vi "Prepare Acquired Waveforms for Parsing.vi"(4 "append virtual reference":bool, 6 "propagation delay":T1, 7 "restart (F)":bool, 8 "error in":errorcluster, 9 "SV Signal":refnum<class "SV Signal.lvclass">, 10 "tolerance":dbl=0.1 format="%#_13g", 11 "acquired channel waveforms":waveform(dbl)[](array[waveform])) -> (0 "error out":errorcluster, 3 "aligned channel waveforms":waveform(dbl)[](array[waveform]), 5 "alignment reference detected":bool)   [LabVIEW 2022 SP3]
doc: "Align signals and optionally append virtual reference prior to writing data to SV Buffer and parsing for measurement samples."
uses:
  <vilib>/addons/_NISVFA/_Generation/Signal Generation/SV Signal/SV Signal.lvclass
  <vilib>/addons/_NISVFA/_Generation/Signal Generation/SV Signal/SV Signal.lvclass/SV Signal.ctl
  <vilib>/addons/_NISVFA/_Generation/Signal Generation/SV Signal/Read Synchronization Pulse Waveform.vi
  Program Files/NI/LVAddons/nisvt/1/examples/Sound and Vibration/Audio Measurements/subVIs/sv_Measure Delay for Active and Idle Channels.vi
  <vilib>/addons/_NISVFA/_Generation/Signal Generation/SV Signal/Read Leading Synchronization Pulse Enable.vi
  <vilib>/addons/_NISVFA/_Generation/Signal Generation/SV Signal/Read Trailing Synchronization Pulse Enable.vi
  <vilib>/addons/_NISVFA/_Generation/Signal Generation/SV Signal/Write Leading Synchronization Pulse Enable.vi
  <vilib>/addons/_NISVFA/_Shared subVIs/Common/svc_Check for Waveform Parameter Continuity (no state).vi
  <vilib>/addons/_NISVFA/_Shared subVIs/Common/sv_Get NI Property Name String.vi
  <vilib>/addons/Sound and Vibration/svt_Calibration/SV Measure Delay and Polarity and Coherence (Nx1).vi
  Program Files/NI/LVAddons/nisvt/1/examples/Sound and Vibration/Audio Measurements/subVIs/sv_Assign Delay to Idle Channels.vi
  <vilib>/addons/_NISVFA/_Shared subVIs/Common/svc_Get SV Channel Info.vi
  <vilib>/addons/Sound and Vibration/svt_Calibration/SV Measure Delay and Polarity and Coherence.vi
  <vilib>/addons/_NISVFA/_Shared subVIs/Common/svc_Unit Label to Engineering Units.vi
  <vilib>/addons/_NISVFA/_Shared subVIs/Common/svc_Engineering Units to Unit Label.vi
  <vilib>/Analysis/_algsub.llb/Vector Norm.vi
  <vilib>/Analysis/_algsub.llb/Real Vector Norm.vi
  <vilib>/addons/_NISVFA/_Shared subVIs/Common/SV Get Data Subset.vi
  <vilib>/addons/_NISVFA/_Shared subVIs/Common/svc_Get Array Subset (Index).vi
  <vilib>/addons/_NISVFA/_Shared subVIs/Common/svc_Coerce Index and Length.vi
  <vilib>/addons/_NISVFA/_Shared subVIs/Common/svc_Conditional Merge Error.vi
  <vilib>/addons/_NISVFA/_Generation/Signal Generation/SV Signal/Read System Timing Model.vi
  <vilib>/addons/_NISVFA/_Generation/Signal Generation/SV Signal/Write System Timing Model.vi
  <vilib>/addons/_NISVFA/_Shared subVIs/Data Objects/Waveforms (DBL)/Write to Buffer.vi
  <vilib>/addons/_NISVFA/_Shared subVIs/Data Objects/Waveforms (DBL)/Read from Buffer.vi
  <vilib>/addons/_NISVFA/_Shared subVIs/Data Objects/Waveforms (DBL)/SV Read Newest Data.vi
  <vilib>/measure/maresamp.llb/Resample Waveforms (single shot).vi
  <vilib>/measure/maresamp.llb/Resample Waveform (single shot).vi
  <vilib>/addons/_NISVFA/_Shared subVIs/Common/svc_Check dt for Equal Sample Rates.vi
  <vilib>/Waveform/TSOps.llb/Timestamp Subtract.vi
  <vilib>/Analysis/2dsp.llb/CrossCorrelation.vi
  <vilib>/Analysis/2dsp.llb/1D Cross Correlation (DBL).vi
  <vilib>/addons/_NISVFA/_Shared subVIs/Common/svc_Fit Quadratic to Max Three Points in Array.vi
  <vilib>/Utility/error.llb/Error Cluster From Error Code.vi
  <vilib>/addons/_NISVFA/_Shared subVIs/Common/svc_Caller VI Returned in Error Source.vi
  <vilib>/addons/_NISVFA/_Shared subVIs/Common/SV Remove Delays (1,N) from Waveforms (N Ch) (DBL).vi
  <vilib>/addons/_NISVFA/_Generation/Signal Generation/SV Signal/Read Sample Rate.vi
  Program Files/NI/LVAddons/nisvt/1/examples/Sound and Vibration/SoundVib_Audio Examples.lvlib
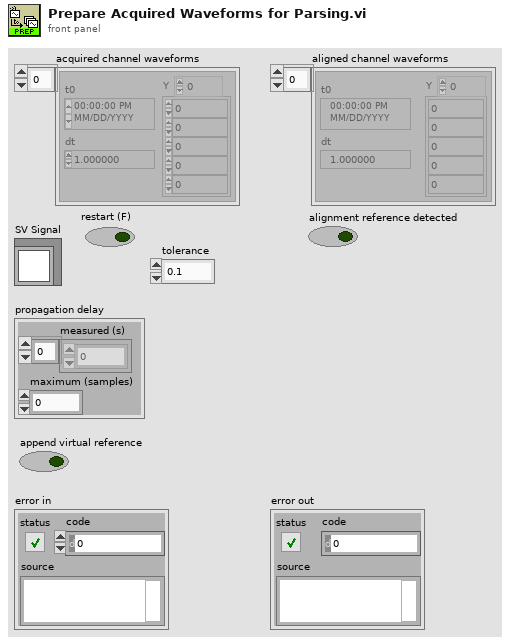
[diagram p1: front panel]
types:
  T1 = cluster{"measured (s)":dbl[], "maximum (samples)":i32}
  T2 = cluster{"dt equal":bool, "array length equal":bool, "number channels change":bool}
  T3 = cluster{"dt":bool, "t0 continuity":bool, "array length":bool, "channel info":bool, "name":bool}
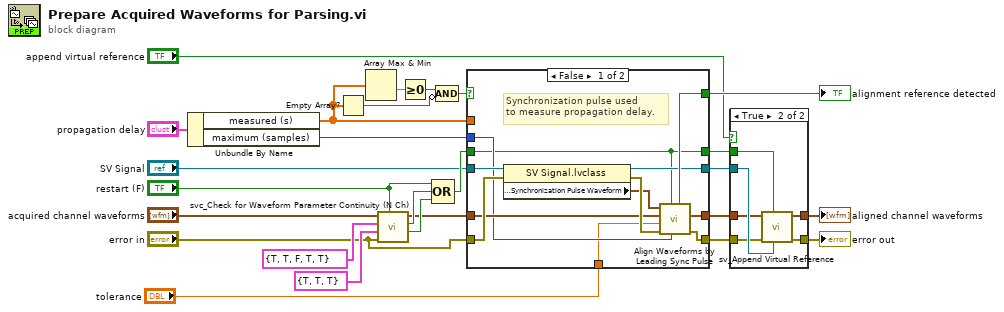
[diagram p0: block diagram]
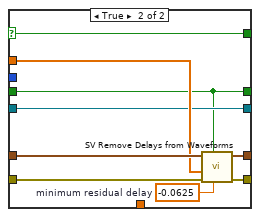
[diagram p3: hidden frame]
diagram:
  n1 = Unbundle By Name("propagation delay") -> ("measured (s)"=w26:dbl[], "maximum (samples)"=w3:i32)
  n2 = Empty Array?(array=w26) -> (empty?=w4:bool)
  n3 = Array Max & Min(array=w26) -> (min value=w23:dbl)  [unwired: 3 out]
  n4 = call <vilib>:"svc_Check for Waveform Parameter Continuity (N Ch).vi"("restart averaging (F)"="restart (F)", "error in"="error in", "checks for multichannel parameters"=T2 {"dt equal"=TRUE, "array length equal"=TRUE, "number channels change"=TRUE}, "checks for channel parameter change"=T3 {"dt"=TRUE, "t0 continuity"=TRUE, "array length"=FALSE, "channel info"=TRUE, "name"=TRUE}, "scaled signal(s)"="acquired channel waveforms") -> ("multichannel parameter changed"=w18:bool, "waveform parameter changed"=w19:bool, "dup scaled signal(s)"=w9:waveform(dbl)[])  [unwired: 4 out]
  n5 = Greater Or Equal To 0?(x=w23) -> (x >= 0?=w24:bool)
  n6 = Compound Arithmetic op=OR("restart (F)", w19, w18) -> (w20:bool)
  n7 = Compound Arithmetic op=AND(w24, invert w4) -> (w25:bool)
  n8 = case shown="False" w25 {
    selector: w25 -> [_ w43]
    tunnel: "error in" -> [w37 w45]
    tunnel: w9 -> [w36 w47]
    tunnel: "SV Signal" -> [w34 w41]
    tunnel: [w33 w44] -> w12
    tunnel: [w32 w46] -> w13
    tunnel: w26 -> [_ w42]
    tunnel: w3 -> [w31 _]
    tunnel: w20 -> [w28 w40]
    tunnel: [w30 w43] -> w22
    tunnel: [w29 w41] -> w8
    tunnel: [w28 w40] -> w7
    tunnel: "tolerance" -> [w27 _]
    frame False {
      # "Synchronization pulse used \nto measure propagation delay."
      n9 = property on="Property Node" class="SV Signal.lvclass"(reference=w34, error in=w37) -> (reference out=w29:refnum<class "SV Signal.lvclass">, error out=w38:errorcluster, "Signal Properties:Synchronization Pulses:Synchronization Pulse Waveform"=w35:waveform(dbl))
      n10 = call "Align Waveforms by Leading Sync Pulse.vi"("maximum delay"=w31, "reset"=w28, "error in (no error)"=w38, "tolerance"=w27, "response signals"=w36, "alignment reference signal"=w35) -> ("error out"=w33:errorcluster, "aligned signals"=w32:waveform(dbl)[], "alignment reference detected"=w30:bool)  [unwired: 1 in, 2 out]
    }
    frame True {
      w39 = -0.0625  # minimum residual delay
      n11 = call-poly <vilib>:"SV Remove Delays from Waveforms.vi"("minimum residual delay"=w39, "reset"=w40, "error in (no error)"=w45, "path-dependent analog delays [s]"=w42, "scaled signals"=w47) -> ("error out"=w44:errorcluster, "aligned signals"=w46:waveform(dbl)[])  [unwired: 3 in, 2 out]
    }
  }
  "alignment reference detected" <- w22
  n12 = case shown="True" "append virtual reference" {
    tunnel: [w49 w55] -> w6
    tunnel: w8 -> [_ w54]
    tunnel: [w48 w53] -> w5
    tunnel: w13 -> [w49 w52]
    tunnel: w12 -> [w48 w51]
    tunnel: w7 -> [_ w50]
    frame False {
    }
    frame True {
      n13 = call "sv_Append Virtual Reference.vi"("SV Signal in"=w54, "reset"=w50, "error in (no error)"=w51, "acquired waveforms"=w52) -> ("error out"=w53:errorcluster, "acquired waveforms with virtual reference"=w55:waveform(dbl)[])  [unwired: 6 in]
    }
  }
  "aligned channel waveforms" <- w6
  "error out" <- w5
